vi "Operate.vi"(8 "error in (no error)":errorcluster, 11 "Arithmetic in":refnum<class "Arithmetic.lvclass">) -> (0 "error out":errorcluster, 2 "C":dbl, 3 "Arithmetic out":refnum<class "Arithmetic.lvclass">)   [LabVIEW 2023, in "Arithmetic.lvclass"]
uses:
  Arithmetic.lvclass
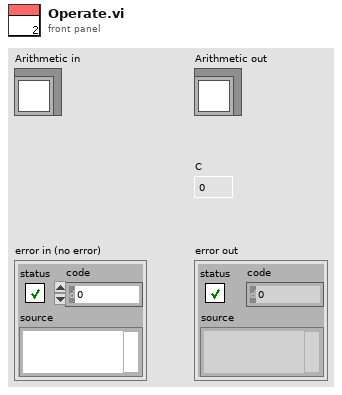
[diagram p1: front panel]
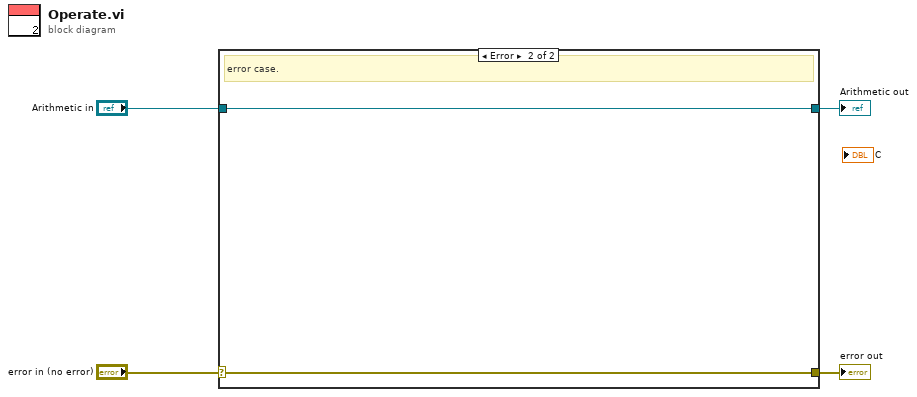
[diagram p0: block diagram]
diagram:
  n1 = case shown="Error" "error in (no error)" {
    selector: "error in (no error)" -> [w5 w8]
    tunnel: [w5 w8] -> w3
    tunnel: [w6 w7] -> w1
    tunnel: "Arithmetic in" -> [w6 w7]
    frame No Error {
      # "Wire the error cluster across even in the \"No Error\"\ncase so that warnings get propagated."
      # "No error case."
    }
    frame Error {
      # "error case."
    }
  }
  "error out" <- w3
  "Arithmetic out" <- w1
